vi "DSF.Engine.Interface.Builder.New.vi"(7 "fifo depths (10)":u32=10, 8 "error in (no error)":errorcluster, 11 "Builder Interface type":refnum<class "DSF.Engine.Interface.Builder.lvclass">) -> (0 "error out":errorcluster, 3 "Builder Interface":refnum<class "DSF.Engine.Interface.Builder.lvclass">)   [LabVIEW 2016, in "DSF.Engine.lvlib" / "DSF.Engine.Interface.Builder.lvclass"]
uses:
  DSF.Engine.Interface.Builder.lvclass
  C:/Git/Sourcetree/DSF/Source/Engine/Classes/Interface/DSF.Engine.Interface.lvclass
  DSF.Engine.Interface.lvclass
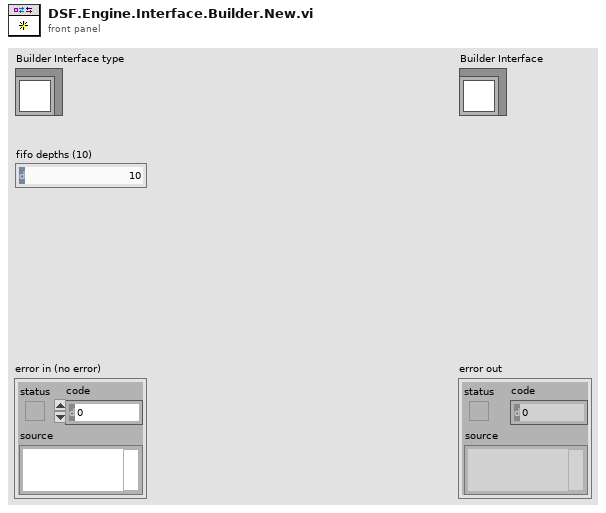
[diagram p1: front panel]
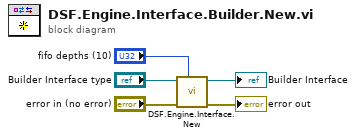
[diagram p0: block diagram]
diagram:
  n1 = call "DSF.Engine.Interface.New.vi"("fifo depths (10)"="fifo depths (10)", "error in (no error)"="error in (no error)", "Interface type"="Builder Interface type") -> ("error out"=→"error out":errorcluster, "Interface"=→"Builder Interface":refnum<class "DSF.Engine.Interface.Builder.lvclass">)  [unwired: 7 in]
